vi "Target.vi"() -> ()   [LabVIEW 2025]
uses:
  <vilib>/Platform/TimedLoop/XDataNode/timing_clust.ctl
  <vilib>/Platform/TimedLoop/XDataNode/nitl_modes.ctl
  <vilib>/Platform/TimedLoop/XDataNode/wakeup.ctl
  <vilib>/rvi/Emulation/niFpgaSctlEmulationGetInTimedLoop.vi
  <vilib>/rvi/Emulation/niFpgaEmulationReportErrorSimple.vi
  <vilib>/rvi/Emulation/niFpgaGetClockAttributes.vi
  <vilib>/rvi/Emulation/niFpgaCriticalErrorInLSC.vi
  <vilib>/rvi/linearAlgebra/MatrixMultiply/simVIs/SubVI/nifxpla_MatrixMultiply_SimMatrixSizes.vi
  <vilib>/rvi/linearAlgebra/MatrixMultiply/simVIs/SubVI/nifxpla_MatrixMultiply_Sim4WireAdapterVector.vi
  <vilib>/rvi/linearAlgebra/MatrixMultiply/simVIs/SubVI/nifxpla_MatrixMultiply_SimFrameHandShake.vi
  <vilib>/rvi/linearAlgebra/MatrixMultiply/simVIs/SubVI/nifxpla_MatrixMultiply_SimEndlessCounter.vi
  <vilib>/rvi/linearAlgebra/MatrixMultiply/simVIs/SubVI/nifxpla_MatrixMultiply_SimVectorDataBuffer.vi
  <vilib>/rvi/ClientSDK/Core/DevComputerLib/Private/Multiply(dfxp64).vi
  <vilib>/rvi/ClientSDK/Core/DevComputerLib/Private/Dfxp128ToDfxp256.vi
  <vilib>/rvi/ClientSDK/Core/DevComputerLib/Private/Add(dfxp256).vi
  <vilib>/rvi/ClientSDK/Core/DevComputerLib/Private/Subtract(dfxp256).vi
  <vilib>/rvi/ClientSDK/Core/DevComputerLib/Private/ToDfxp64(dfxp256).vi
  <vilib>/platform/TimedLoop/XDataNode/XDataNode.xnode
  <vilib>/rvi/linearAlgebra/MatrixMultiply/XNode/nifxpla_MatrixMultiply.xnode
  <vilib>/rvi/linearAlgebra/MatrixMultiply/simVIs/nifxpla_MatrixMultiply_SimTemplateEinEout.vi
  <vilib>/rvi/linearAlgebra/MatrixMultiply/simVIs/nifxpla_MatrixMultiply_SimTemplateEinVout.vi
  <vilib>/rvi/linearAlgebra/MatrixMultiply/simVIs/nifxpla_MatrixMultiply_SimTemplateVinEout.vi
  <vilib>/rvi/linearAlgebra/MatrixMultiply/simVIs/nifxpla_MatrixMultiply_SimTemplateVinVout.vi
  <vilib>/Platform/TimedLoop/XDataNode/XDNodeRunTimeDep.lvlib
panel:
  out "Array 2":fxp<+/-,32,16>[](array[numeric])
  out "Array":fxp<+/-,32,16>[](array[numeric])
  out "Numeric":i32
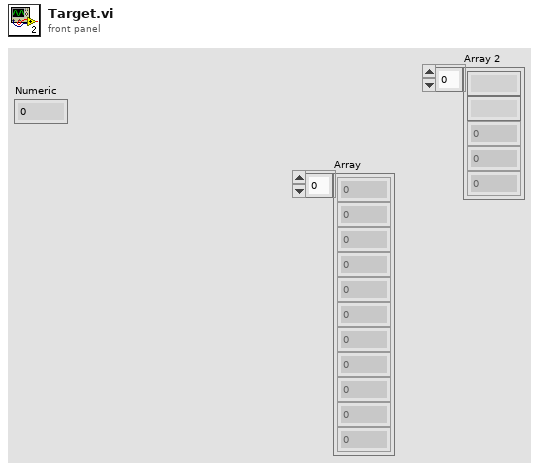
[diagram p1: front panel]
types:
  T1 = typedef "XDNodeRunTimeDep.lvlib/timing_clust.ctl" = cluster{"Expected End [f-1]":u64, "Actual End [f-1]":u64, "Finished Late? [f-1]":bool, "Expected End [i-1]":u64, "Actual End [i-1]":u64, "Finished Late? [i-1]":bool, "Expected Start [i]":u64, "Actual Start [i]":u64, "Expected Start [f]":u64, "Actual Start [f]":u64, "Source Name":string, "Structure Name":string, "Period":i64, "Deadline":i64, "Offset":i64, "Start":i64, "Priority":i32, "Timeout":i32, "Mode":T2, "Wakeup Reason":T3, "Error":errorcluster, "Source Type":string, "Secondary Source Type":string, "Global End Time":u64, "Global Start Time":u64, "Frame Duration":u64, "Iteration Duration":u64, "Assigned CPU":i32, "I/O Scan Engine Mode":u32}
  T2 = typedef "XDNodeRunTimeDep.lvlib/nitl_modes.ctl" = enum32{"No Change", "Process missed periods, maintain original phase", "Discard missed periods, maintain original phase", "Process missed periods, ignore original phase", "Discard missed periods, ignore original phase"}
  T3 = typedef "XDNodeRunTimeDep.lvlib/wakeup.ctl" = enum32{"Normal", "Aborted", "Asynchronous wakeup", "Timing source error", "Timed loop error", "Timeout"}
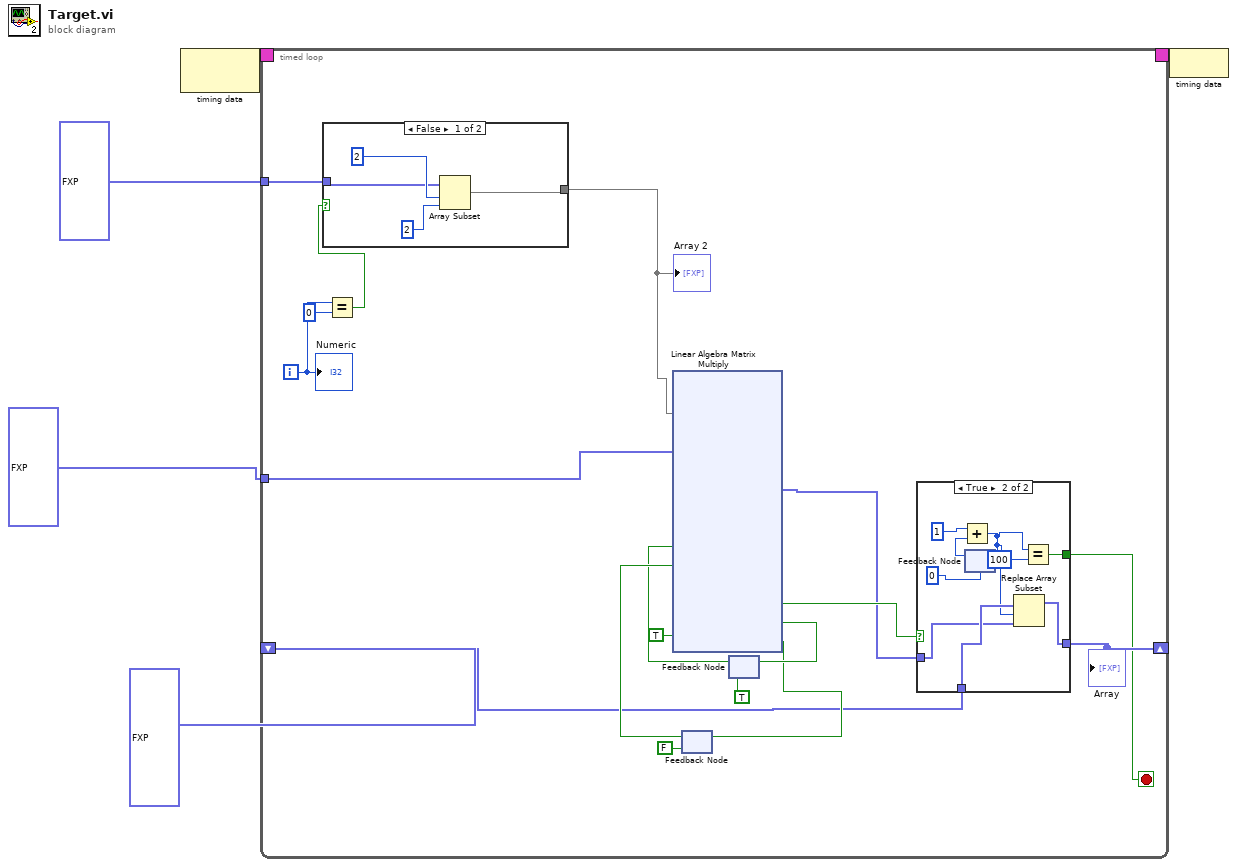
[diagram p0: block diagram]
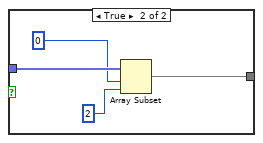
[diagram p2: hidden frame]
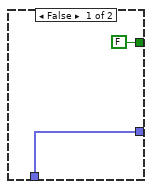
[diagram p3: hidden frame]
diagram:
  n1 = node-c288() -> (w5:T1)  [unwired: 1 in]
  n2 = timed-loop {
    timing: w5 -> [_]
    timing-out: [_] -> w4
    shift-right: [w15] -> _
    shift-left: fxp<+/-,32,16>[] [0.0, 0.0, 0.0, 0.0, 0.0, 0.0, 0.0] -> [w14]
    tunnel: fxp<+/-,32,16>[] [1.0, 2.0] -> [w12]
    tunnel: fxp<+/-,32,16>[] [1.0, 2.0, 3.0, 4.0] -> [w10]
    i -> [w8]
    stop <- w13 stop-if-true
    n3 = Equal?(x=w8, y=0) -> (x = y?=w6:bool)
    n4 = case shown="False" w6 {
      tunnel: w10 -> [w25 w31]
      tunnel: [w24 w29] -> w9
      frame False {
        n5 = Array Subset(array=w25, index=2 ("length"), length=2) -> (w24:fxp<+/-,32,16>[])
      }
      frame True {
        n6 = Array Subset(array=w31, index=0 ("length"), length=2) -> (w29:fxp<+/-,32,16>[])
      }
    }
    "Array 2" <- w9
    n7 = feedback #1(FALSE ("ready for b")) -> (w21:bool)
    n8 = feedback #2(TRUE ("ready for a")) -> (w11:bool)
    n9 = xnode ("Linear Algebra Matrix Multiply")("ar"=w9, "br"=w12, "a valid"=w11, "b valid"=w21, "ready for output (T)"=TRUE) -> ("cr"=w16:fxp<+/-,32,16>[], "output valid"=w17:bool, "ready for a"=w23:bool, "ready for b"=w22:bool)  [unwired: 2 in, 2 out]
    n10 = feedback-in #1(w22) -> ()
    n11 = feedback-in #2(w23) -> ()
    n12 = case shown="True" w17 {
      tunnel: w16 -> [_ w34]
      tunnel: [w33 w41] -> w15
      tunnel: w14 -> [w33 w42]
      tunnel: [FALSE w35] -> w13
      frame False {
      }
      frame True {
        n13 = feedback #3(0 ("x")) -> (w39:i32)
        n14 = Add(x=1, y=w39) -> (x+y=w37:i32)
        n15 = feedback-in #3(w37) -> ()
        n16 = Replace Array Subset(array=w42, new element=w34, index=w37) -> (w41:fxp<+/-,32,16>[])
        n17 = Equal?(x=w37, y=100) -> (x = y?=w35:bool)
      }
    }
    "Array" <- w15
    "Numeric" <- w8
  }
  n18 = node-c288(w4) -> ()
